vi "get set names.vi"(8 "error in (no error)":errorcluster, 11 "manager_daemon in":refnum<class "manager_daemon.lvclass">) -> (0 "error out":errorcluster, 2 "set names":T1, 3 "manager_daemon out":refnum<class "manager_daemon.lvclass">)   [LabVIEW 2024, in "manager_daemon.lvclass"]
uses:
  manager_daemon.lvclass
  manager_daemon.lvclass/manager_daemon.ctl
  type_defs/cmd--enum.ctl
  type_defs/msg--cluster.ctl
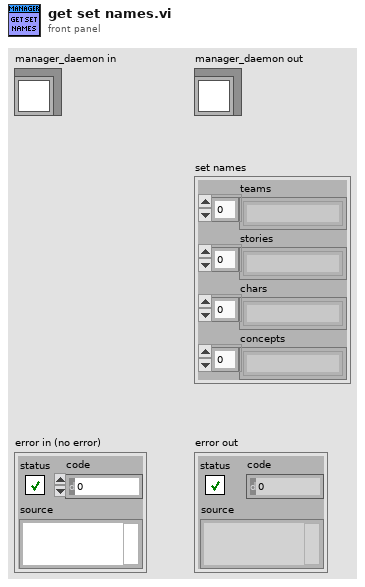
[diagram p1: front panel]
types:
  T1 = cluster{"teams":string[], "stories":string[], "chars":string[], "concepts":string[]}
  T2 = typedef "manager_daemon.lvclass/cmd--enum.ctl" = enum16{"init", "run", "load binaries", "save binaries", "updated volume", "get set names", "return vol path by id", "return vol ids by publisher", "display info", "filter release week", "apply filter", "add publisher", "get publishers", "add volume", "add issues", "add issue", "delete volume", "delete issues", "download issues", "exit"}
  T3 = typedef "manager_daemon.lvclass/msg--cluster.ctl" = cluster{"cmd":T2, "data":variant}
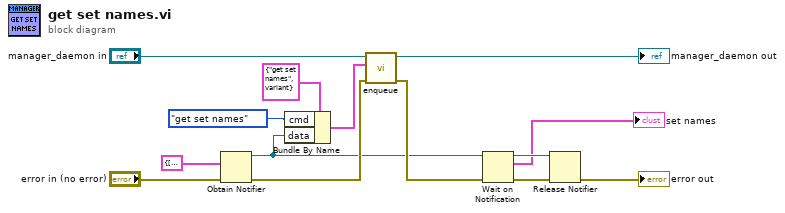
[diagram p0: block diagram]
diagram:
  n1 = Obtain Notifier(notification data type=T1 {"teams"=[], "stories"=[], "chars"=[], "concepts"=[]}, error in (no error)="error in (no error)") -> (notifier out=w6:refnum<notifier>, error out=w9:errorcluster)  [unwired: 2 in, 1 out]
  n2 = Bundle By Name(cluster=T3 {"cmd"=enum."get set names", "data"=variant} ("msg"), "cmd"=cmd--enum."get set names", "data"=w6) -> (w11:T3)
  n3 = call "enqueue.vi"("error in (no error)"=w9, "msg"=w11, "manager_daemon in"="manager_daemon in") -> ("error out"=w7:errorcluster, "manager_daemon out"=→"manager_daemon out":refnum<class "manager_daemon.lvclass">)  [unwired: 7 in]
  n4 = Wait on Notification(notifier=w6, error in (no error)=w7) -> (notifier out=w2:refnum<notifier>, notification=→"set names":T1, error out=w4:errorcluster)  [unwired: 2 in, 1 out]
  n5 = Release Notifier(notifier=w2, error in (no error)=w4) -> (error out=→"error out":errorcluster)  [unwired: 1 in, 2 out]
